vi "clone.vi"(0 "reference":refnum<class "NoteEdge.lvclass">, 5 "error in (no error)":errorcluster) -> (14 "reference out":refnum<class "NoteEdge.lvclass">, 15 "clonedNoteEdge":refnum<class "AbstractEdge.lvclass">, 19 "error out":errorcluster)   [LabVIEW 2020, in "NoteEdge.lvclass"]
doc: "Clone object"
uses:
  <resource>/Framework/Providers/Open_GDS/UML/NoteEdge_class/NoteEdge.lvclass
  C:/Program Files (x86)/National Instruments/LabVIEW 2020/resource/Framework/Providers/Open_GDS/UML/GeneralPathEdge_class/GeneralPathEdge.lvclass
  C:/Program Files (x86)/National Instruments/LabVIEW 2020/resource/Framework/Providers/Open_GDS/UML/AbstractEdge_class/AbstractEdge.lvclass
  <resource>/Framework/Providers/Open_GDS/UML/AbstractEdge_class/AbstractEdge.lvclass
  <resource>/Framework/Providers/Open_GDS/UML/GeneralPathEdge_class/GeneralPathEdge.lvclass
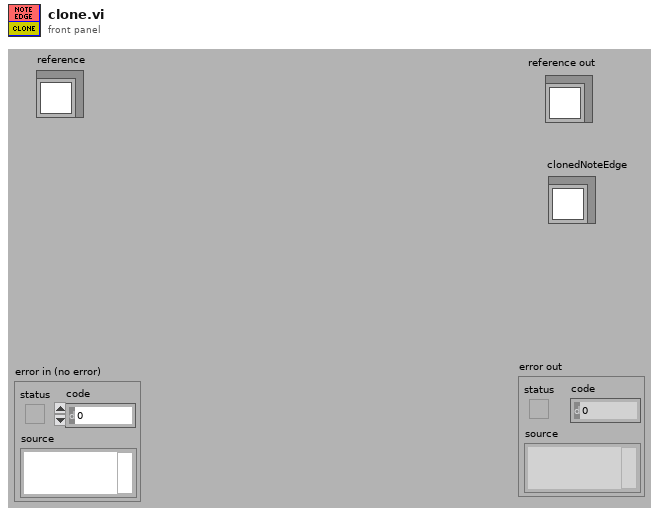
[diagram p1: front panel]
types:
  T1 = typedef "NoteEdge.lvclass/ObjectAttributes.ctl" = cluster{"None":bool}
  T2 = typedef "GeneralPathEdge.lvclass/ObjectAttributes.ctl" = cluster{"None":bool}
  T3 = typedef "AbstractEdge.lvclass/ObjectAttributes.ctl" = cluster{"start":refnum<class "AbstractNode.lvclass">, "end":refnum<class "AbstractNode.lvclass">}
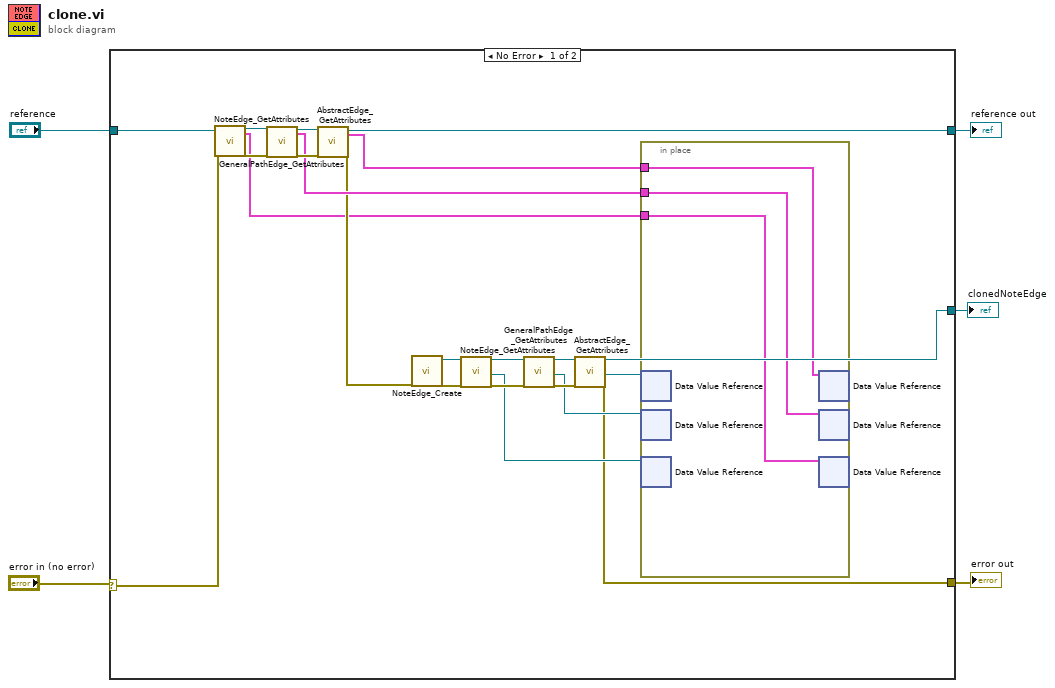
[diagram p0: block diagram]
diagram:
  n1 = case shown="No Error" "error in (no error)" {
    selector: "error in (no error)" -> [w16 w31]
    tunnel: "reference" -> [w18 w32]
    tunnel: [w7 w31] -> w4
    tunnel: [w6 w32] -> w3
    tunnel: [w8 _] -> w1
    frame No Error {
      n2 = call <resource>:"NoteEdge_GetAttributes.vi"("reference in"=w18, "error in (no error)"=w16) -> ("reference out"=w17:refnum<class "NoteEdge.lvclass">, "Data"=w9:T1, "error out"=w19:errorcluster)  [unwired: 14 in, 1 out]
      n3 = call <resource>:"GeneralPathEdge_GetAttributes.vi"("reference in"=w17, "error in (no error)"=w19) -> ("reference out"=w27:refnum<class "NoteEdge.lvclass">, "Data"=w23:T2, "error out"=w26:errorcluster)  [unwired: 14 in, 1 out]
      n4 = call <resource>:"AbstractEdge_GetAttributes.vi"("reference in"=w27, "error in (no error)"=w26) -> ("reference out"=w6:refnum<class "NoteEdge.lvclass">, "Data"=w22:T3, "error out"=w15:errorcluster)  [unwired: 14 in, 1 out]
      n5 = call <resource>:"NoteEdge_Create.vi"("error in (no error)"=w15) -> ("reference out"=w14:refnum<class "NoteEdge.lvclass">, "error out"=w13:errorcluster)  [unwired: 17 in]
      n6 = call <resource>:"NoteEdge_GetAttributes.vi"("reference in"=w14, "error in (no error)"=w13) -> ("reference out"=w12:refnum<class "NoteEdge.lvclass">, "DataRef"=w10:refnum<data-value>, "error out"=w11:errorcluster)  [unwired: 14 in, 1 out]
      n7 = call <resource>:"GeneralPathEdge_GetAttributes.vi"("reference in"=w12, "error in (no error)"=w11) -> ("reference out"=w24:refnum<class "NoteEdge.lvclass">, "DataRef"=w20:refnum<data-value>, "error out"=w25:errorcluster)  [unwired: 14 in, 1 out]
      n8 = call <resource>:"AbstractEdge_GetAttributes.vi"("reference in"=w24, "error in (no error)"=w25) -> ("reference out"=w8:refnum<class "NoteEdge.lvclass">, "DataRef"=w21:refnum<data-value>, "error out"=w7:errorcluster)  [unwired: 14 in, 1 out]
      n9 = in-place {
        in-place-border: w9 -> [w30]
        in-place-border: w23 -> [w29]
        in-place-border: w22 -> [w28]
        n10 = in-place-dvr #1(w21) -> ()  [unwired: 2 out]
        n11 = in-place-dvr #2(w20) -> ()  [unwired: 2 out]
        n12 = in-place-dvr #3(w10) -> ()  [unwired: 2 out]
        n13 = in-place-dvr #1(w28) -> ()  [unwired: 2 out]
        n14 = in-place-dvr #2(w29) -> ()  [unwired: 2 out]
        n15 = in-place-dvr #3(w30) -> ()  [unwired: 2 out]
      }
    }
    frame Error {
    }
  }
  "reference out" <- w3
  "error out" <- w4
  "clonedNoteEdge" <- w1
